vi "logger.vi"(8 "error in (no error)":errorcluster, 11 "module name":string="log") -> (0 "error out":errorcluster)   [LabVIEW 2019]
uses:
  common/common data types/common_event_data.ctl
panel:
  out "log":string
  out "global stop?":bool
  out "data":variant
  in  "stop this module":bool
  out "targetted":bool
  out "target":string
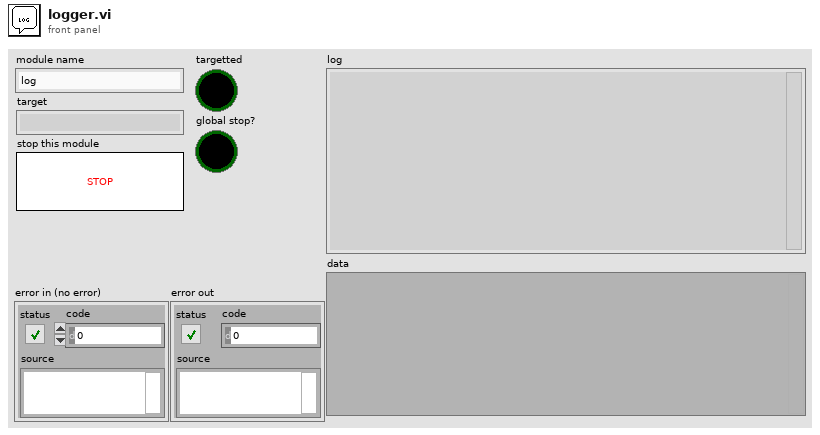
[diagram p1: front panel]
types:
  T1 = typedef "common_event_data.ctl" = cluster{"sender":string, "target":string, "msg":string, "data":variant}
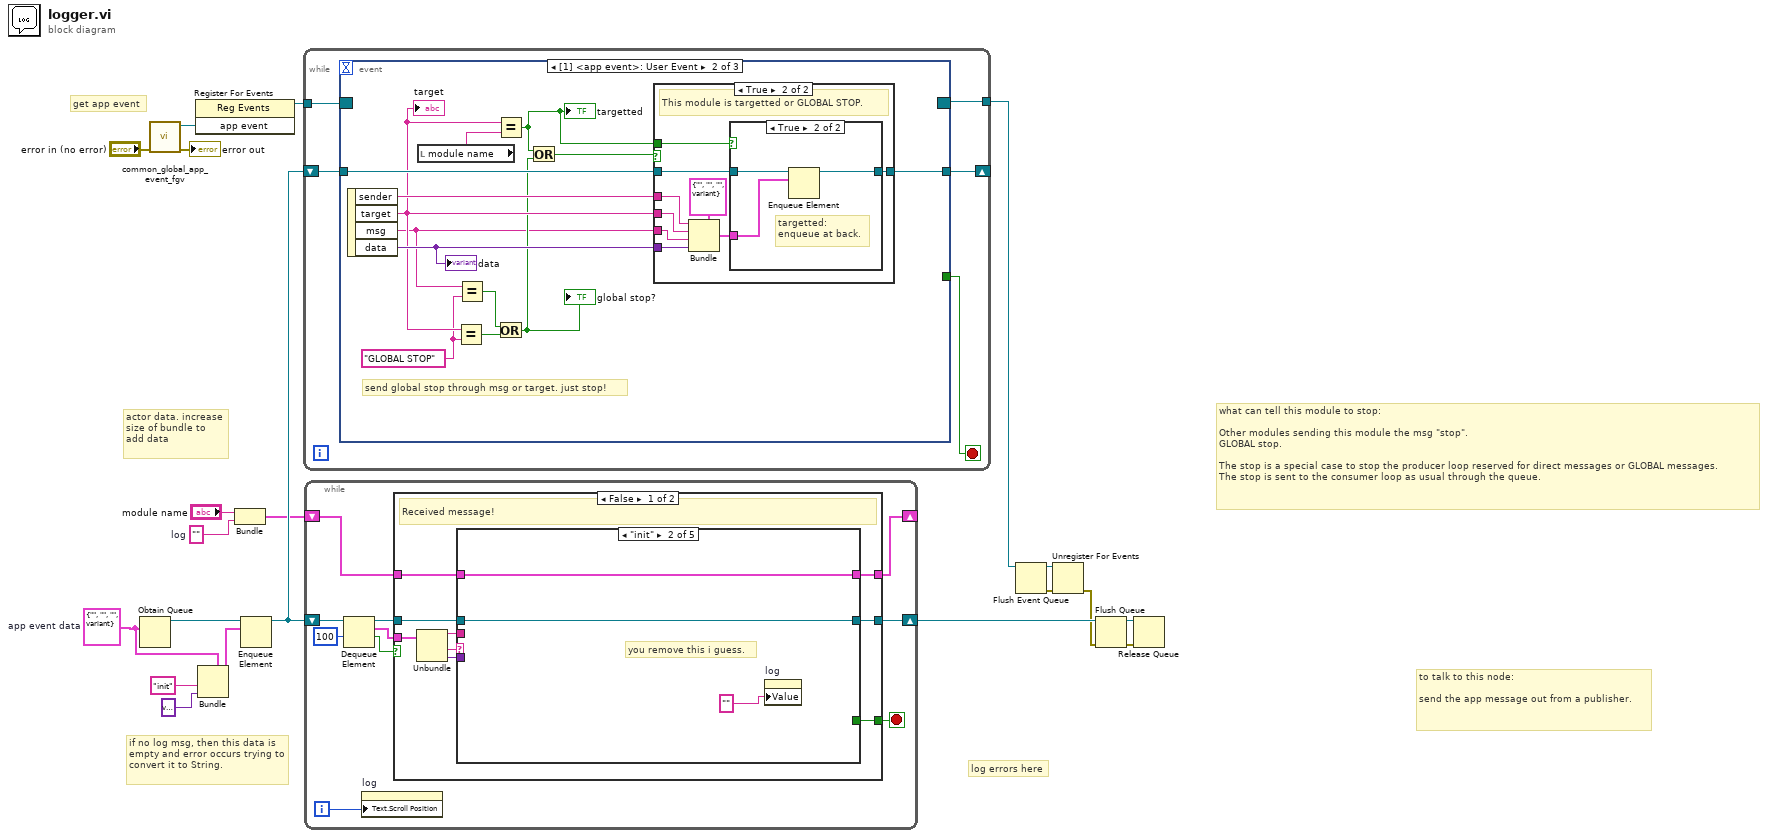
[diagram p0: block diagram]
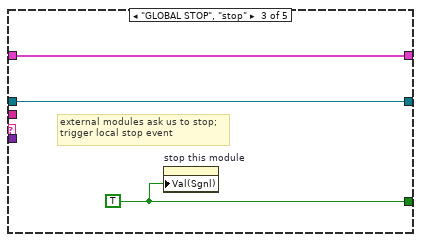
[diagram p3: hidden frame]
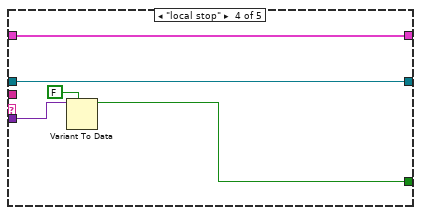
[diagram p4: hidden frame]
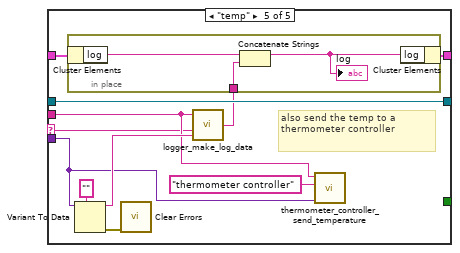
[diagram p5: hidden frame]
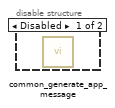
[diagram p7: hidden frame]
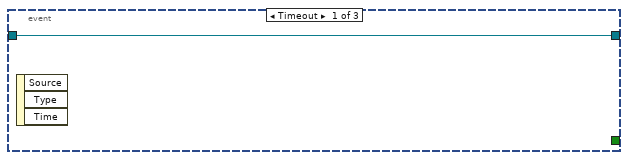
[diagram p8: hidden frame]
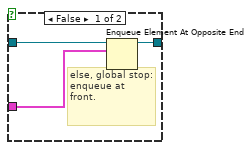
[diagram p10: hidden frame]
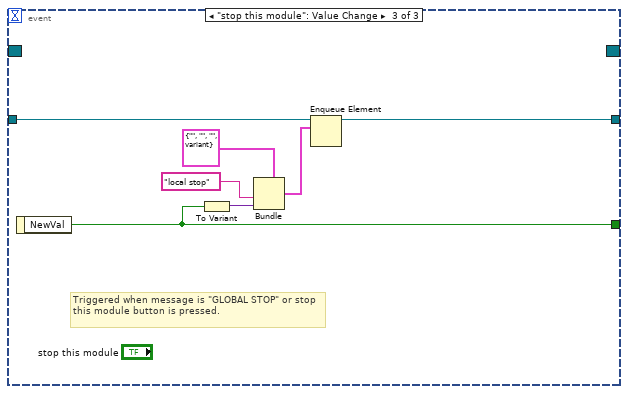
[diagram p11: hidden frame]
diagram:
  w5 = ""  # log
  w9 = T1 {"sender"="", "target"="", "msg"="", "data"=variant}  # app event data
  # "if no log msg, then this data is empty and error occurs trying to convert it to String."
  # "log errors here"
  # "actor data. increase size of bundle to add data"
  # "to talk to this node:\n\nsend the app message out from a publisher."
  # "what can tell this module to stop:\n\nOther modules sending this module the msg \"stop\".\nGLOBAL stop.\n\nThe stop is a special case to stop the producer loop reserved for direct messages or GLOBAL messages.\nThe stop is sent to the consumer loop as usual through the queue."
  # "get app event"
  n1 = Obtain Queue(element data type=w9) -> (queue out=w20:refnum<queue>)  [unwired: 4 in, 2 out]
  n2 = call "common_global_app_event_fgv.vi"("error in (no error)"="error in (no error)") -> ("error out"=→"error out":errorcluster, "app event"=w14:refnum<user-event>)  [unwired: 9 in]
  n3 = register-events(w14) -> (reference out=w15:refnum<event-registration>)  [unwired: 2 in, 1 out]
  n4 = Bundle(cluster=w9, "msg"="init", "data"=variant) -> (w19:T1)  [unwired: 2 in]
  n5 = Bundle("module name"="module name", "log"=w5) -> (w6:cluster{"module name":string, "log":string})  [unwired: 1 in]
  n6 = Enqueue Element(queue=w20, element=w19) -> (queue out=w18:refnum<queue>)  [unwired: 2 in, 2 out]
  n7 = while {
    tunnel: w15 -> [w25]
    shift-right: [w23] -> _
    shift-left: w18 -> [w24]
    tunnel: [w22] -> w4
    stop <- w21 stop-if-true
    n8 = event shown="[1] <app event>: User Event" {
      selector: w25 -> [_ _ _]
      dyn-events: [_ _ _] -> w22
      timeout: _ -> [_ _ _]
      tunnel: w24 -> [w26 w38 w60]
      tunnel: [w26 w37 w61] -> w23
      tunnel: [_ _ w56] -> w21
      event Timeout {
        n9 = event-data() -> ()  [unwired: 1 in, 3 out]
      }
      event User Event {
        w30 = "GLOBAL STOP"
        # "send global stop through msg or target. just stop!"
        n10 = event-data() -> ("sender"=w36:string, "target"=w35:string, "msg"=w29:string, "data"=w39:variant)  [unwired: 1 in]
        "target" <- w35
        "data" <- w39
        n11 = local read "module name"() -> (w27:string)
        n12 = Equal?(x=w35, y=w30) -> (x = y?=w32:bool)
        n13 = Equal?(x=w29, y=w30) -> (x = y?=w28:bool)
        n14 = Equal?(x=w35, y=w27) -> (x = y?=w33:bool)
        "targetted" <- w33
        n15 = Or(x=w28, y=w32) -> (x .or. y?=w31:bool)
        "global stop?" <- w31
        n16 = Or(x=w33, y=w31) -> (x .or. y?=w34:bool)
        n17 = case shown="True" w34 {
          tunnel: w29 -> [_ w45]
          tunnel: w39 -> [_ w46]
          tunnel: w38 -> [w40 w49]
          tunnel: [w40 w48] -> w37
          tunnel: w35 -> [_ w44]
          tunnel: w36 -> [_ w43]
          tunnel: w33 -> [_ w41]
          frame False {
          }
          frame True {
            # "This module is targetted or GLOBAL STOP."
            n18 = Bundle(cluster=T1 {"sender"="", "target"="", "msg"="", "data"=variant}, "sender"=w43, "target"=w44, "msg"=w45, "data"=w46) -> (w42:T1)
            n19 = case shown="True" w41 {
              tunnel: w49 -> [w50 w55]
              tunnel: [w52 w54] -> w48
              tunnel: w42 -> [w51 w53]
              frame False {
                # "else, global stop: \nenqueue at front."
                n20 = Enqueue Element At Opposite End(queue=w50, element=w51) -> (queue out=w52:refnum<queue>)  [unwired: 2 in, 2 out]
              }
              frame True {
                # "targetted:\nenqueue at back."
                n21 = Enqueue Element(queue=w55, element=w53) -> (queue out=w54:refnum<queue>)  [unwired: 2 in, 2 out]
              }
            }
          }
        }
      }
      event "stop this module": Value Change {
        # "Triggered when message is \"GLOBAL STOP\" or stop this module button is pressed."
        n22 = event-data() -> ("NewVal"=w56:bool)  [unwired: 1 in]
        n23 = To Variant(anything=w56) -> (Variant=w57:variant)
        n24 = Bundle(cluster=T1 {"sender"="", "target"="", "msg"="", "data"=variant}, "msg"="local stop", "data"=w57) -> (w62:T1)  [unwired: 2 in]
        n25 = Enqueue Element(queue=w60, element=w62) -> (queue out=w61:refnum<queue>)  [unwired: 2 in, 2 out]
      }
    }
  }
  n26 = while {
    shift-right: [w69] -> w16
    shift-left: w18 -> [w72]
    shift-right: [w64] -> _
    shift-left: w6 -> [w65]
    i -> [w63]
    stop <- w68 stop-if-true
    n27 = Dequeue Element(queue=w72, timeout in ms (-1)=100) -> (queue out=w70:refnum<queue>, element=w71:T1, timed out?=w67:bool)  [unwired: 1 in, 1 out]
    n28 = property on="log" class="Str"("Text.Scroll Position"=w63) -> ()  [unwired: 2 in, 2 out]
    n29 = case shown="False" w67 {
      tunnel: w71 -> [w81 _]
      tunnel: w70 -> [w80 w110]
      tunnel: [w79 w110] -> w69
      tunnel: [w78 _] -> w68
      tunnel: w65 -> [w75 w109]
      tunnel: [w74 w109] -> w64
      frame False {
        # "Received message!"
        n30 = Unbundle(w81) -> ("sender"=w76:string, "msg"=w73:string, "data"=w77:variant)  [unwired: 1 out]
        n31 = case shown="\"init\"" w73 {
          selector: w73 -> [_ _ _ _ w95]
          tunnel: w80 -> [w83 w86 w89 w94 w105]
          tunnel: [w83 w86 w89 w94 w105] -> w79
          tunnel: w77 -> [_ _ _ w92 w97]
          tunnel: [_ _ w88 w90 _] -> w78
          tunnel: w76 -> [_ _ _ _ w96]
          tunnel: w75 -> [w82 w85 w87 w91 w103]
          tunnel: [w82 w85 w87 w91 w102] -> w74
          frame Default {
          }
          frame "init" {
            # "you remove this i guess."
            n32 = property on="log" class="Str"("Value"="") -> ()  [unwired: 2 in, 2 out]
          }
          frame "GLOBAL STOP", "stop" {
            w88 = TRUE
            # "external modules ask us to stop;\ntrigger local stop event"
            n33 = property on="stop this module" class="Bool (strict)"("Val(Sgnl)"=w88) -> ()  [unwired: 2 in, 2 out]
          }
          frame "local stop" {
            n34 = Variant To Data(type=FALSE, Variant=w92) -> (data=w90:bool)  [unwired: 1 in, 1 out]
          }
          frame "temp" {
            # "also send the temp to a thermometer controller"
            n35 = Variant To Data(type="", Variant=w97) -> (data=w100:string, error out=w101:errorcluster)  [unwired: 1 in]
            n36 = call <vilib>:"Clear Errors.vi"("error in (no error)"=w101) -> ()  [unwired: 5 in, 2 out]
            n37 = call "logger_make_log_data.vi"("Data"=w100, "Msg"=w95, "Sender"=w96) -> ("log data"=w99:string)  [unwired: 1 in]
            n38 = in-place {
              in-place-border: w99 -> [w106]
              n39 = in-place-cluster #1(w103) -> ("log"=w108:string)
              n40 = Concatenate Strings(w108, w106) -> (w107:string)
              "log" <- w107
              n41 = in-place-cluster #1("log"=w107) -> (w102:cluster{"module name":string, "log":string})
            }
            n42 = call "thermometer_controller_send_temperature.vi"("data"=w97, "target (thermometer controller)"="thermometer controller", "sender"=w96) -> ()  [unwired: 9 in]
          }
        }
      }
      frame True {
        # "Timeout is a good place to do periodic items. Use this VI to send them where they need to go."
        # "Did not receive message; timed out."
        n43 = disable-structure shown="Enabled" {
          frame Disabled {
            n44 = call "common_generate_app_message.vi"() -> ()  [unwired: 11 in, 1 out]
          }
          frame Enabled {
          }
        }
      }
    }
  }
  n45 = Flush Event Queue(0:w4) -> (8:w3:refnum<event-registration>, 11:w2:errorcluster)  [unwired: 5 in, 1 out]
  n46 = Unregister For Events(event registration refnum=w3, error in=w2) -> (error out=w11:errorcluster)
  n47 = Flush Queue(queue=w16, error in (no error)=w11) -> (queue out=w17:refnum<queue>, error out=w10:errorcluster)  [unwired: 1 out]
  n48 = Release Queue(queue=w17, error in (no error)=w10) -> ()  [unwired: 1 in, 3 out]
